vi "Start.vi"(6 "ms timeout (if waiting)":i32=-1, 8 "error in (no error)":errorcluster, 9 "Wait Until Shutdown? (F)":bool, 11 "SMO":refnum<class "SMO.lvclass">) -> (0 "error out":errorcluster, 3 "SMO out":refnum<class "SMO.lvclass">)   [LabVIEW 2013, in "SMO.lvclass"]
doc: "In the default mode (when <b>Wait Until Shutdown?</b> is False), this method will start (launch asynchronously) the registered processes.\n\nIf <b>Wait Until Shutdown?</b> is True, then this method is blocking (process launch is synchronous) until either the stop method is invoked or <b>ms timeout</b> is reached.\n\nNote 01: This method is overridable by descendant\nNote 02: When overridden, Call Parent Method is required\n\n---------------------------------------------------------------\nJKI State Machine Objects™\nhttp://jki.net/state-machine-objects/\nCopyright (C) 2005-2015, JKI <info@jki.net>\nALL RIGHTS RESERVED"
uses:
  SMO.lvclass
  Typedefs/SMOState --Enum.ctl
panel:
  # "For instructions on how to use the JKI State Machine Objects, examples and video tutorials, visit:\nhttp://jki.net/state-machine-objects/\n\nJKI State Machine Objects™\nhttp://jki.net/state-machine-objects/\nCopyright (C) 2005-2015, JKI <info@jki.net>\nALL RIGHTS RESERVED"
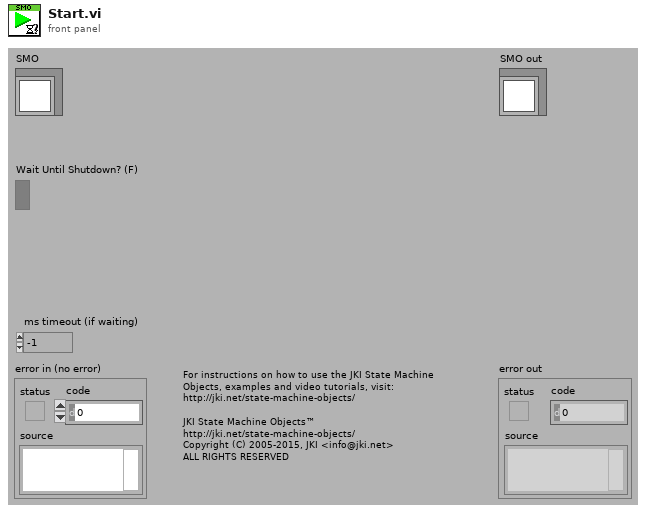
[diagram p1: front panel]
types:
  T1 = typedef "SMO.lvclass/SMOState --Enum.ctl" = enum16{"unknown", "Created", "Started", "Stopped"}
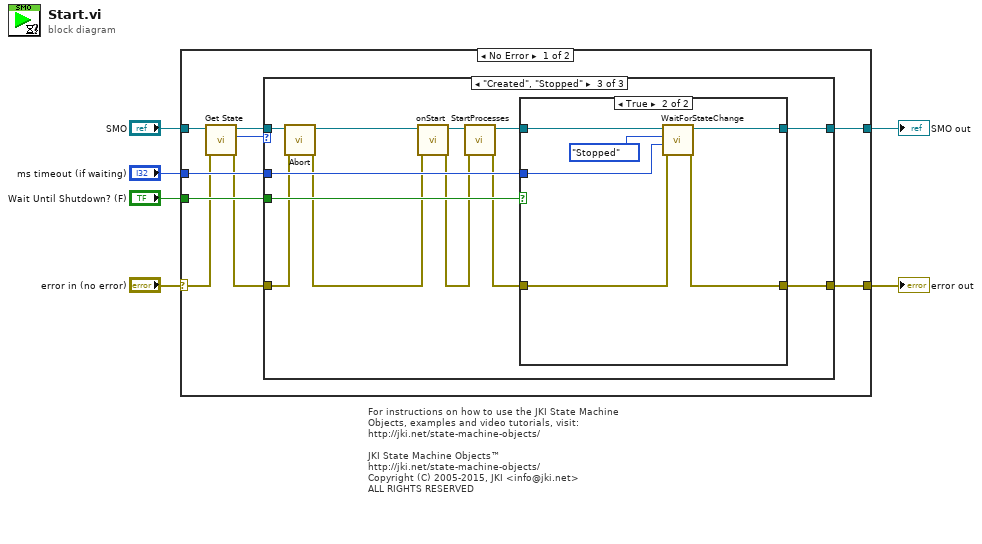
[diagram p0: block diagram]
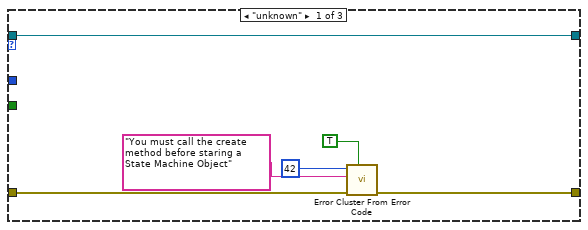
[diagram p2: hidden frame]
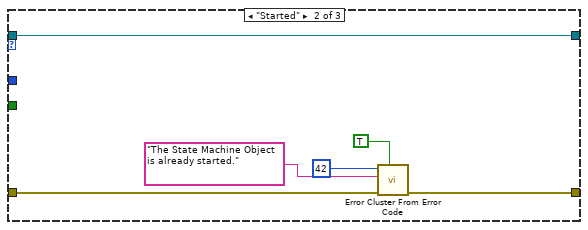
[diagram p3: hidden frame]
diagram:
  # "For instructions on how to use the JKI State Machine Objects, examples and video tutorials, visit:\nhttp://jki.net/state-machine-objects/\n\nJKI State Machine Objects™\nhttp://jki.net/state-machine-objects/\nCopyright (C) 2005-2015, JKI <info@jki.net>\nALL RIGHTS RESERVED"
  n1 = case shown="No Error" "error in (no error)" {
    selector: "error in (no error)" -> [w11 w49]
    tunnel: [w7 w49] -> w5
    tunnel: [w8 w48] -> w3
    tunnel: "SMO" -> [w13 w48]
    tunnel: "Wait Until Shutdown? (F)" -> [w15 _]
    tunnel: "ms timeout (if waiting)" -> [w14 _]
    frame No Error {
      n2 = call "Get State.vi"("error in (no error)"=w11, "SMO"=w13) -> ("error out"=w10:errorcluster, "SMO State"=w9:T1, "SMO out"=w12:refnum<class "SMO.lvclass">)  [unwired: 7 in]
      n3 = case shown="\"Created\", \"Stopped\"" w9 {
        tunnel: [w21 w27 w39] -> w8
        tunnel: [w20 w26 w38] -> w7
        tunnel: w15 -> [_ _ w37]
        tunnel: w14 -> [_ _ w36]
        tunnel: w12 -> [w21 w27 w29]
        tunnel: w10 -> [w17 w23 w28]
        frame "unknown" {
          n4 = call <vilib>:"Error Cluster From Error Code.vi"("show call chain? (False)"=TRUE, "error in (no error)"=w17, "error message (\"\")"="You must call the create method before staring a State Machine Object" ("error message (\"\")"), "error code (0)"=42) -> ("error out"=w20:errorcluster)  [unwired: 5 in]
        }
        frame "Started" {
          n5 = call <vilib>:"Error Cluster From Error Code.vi"("show call chain? (False)"=TRUE, "error in (no error)"=w23, "error message (\"\")"="The State Machine Object is already started." ("error message (\"\")"), "error code (0)"=42) -> ("error out"=w26:errorcluster)  [unwired: 5 in]
        }
        frame "Created", "Stopped" {
          n6 = call "Abort.vi"("error in (no error)"=w28, "SMO"=w29) -> ("error out"=w31:errorcluster, "SMO out"=w33:refnum<class "SMO.lvclass">)  [unwired: 8 in]
          n7 = call-dynamic "onStart.vi"("error in (no error)"=w31, "SMO"=w33) -> ("error out"=w30:errorcluster, "SMO out"=w32:refnum<class "SMO.lvclass">)  [unwired: 8 in]
          n8 = call "StartProcesses.vi"("error in (no error)"=w30, "SMO"=w32) -> ("error out"=w34:errorcluster, "SMO out"=w35:refnum<class "SMO.lvclass">)  [unwired: 8 in]
          n9 = case shown="True" w37 {
            tunnel: w35 -> [w41 w45]
            tunnel: [w41 w44] -> w39
            tunnel: w34 -> [w40 w43]
            tunnel: [w40 w46] -> w38
            tunnel: w36 -> [_ w47]
            frame False {
            }
            frame True {
              n10 = call "WaitForStateChange.vi"("error in (no error)"=w43, "timeout in ms (-1)"=w47, "State (unknown: Any state change)"=SMOState_--Enum."Stopped", "SMO in"=w45) -> ("error out"=w46:errorcluster, "SMO out"=w44:refnum<class "SMO.lvclass">)  [unwired: 5 in, 1 out]
            }
          }
        }
      }
    }
    frame Error {
    }
  }
  "error out" <- w5
  "SMO out" <- w3
